vi "SetRtMode.vi"(8 "错误输入（无错误）":errorcluster, 10 "收发模式":u8) -> (0 "错误输出":errorcluster)   [LabVIEW 2018]
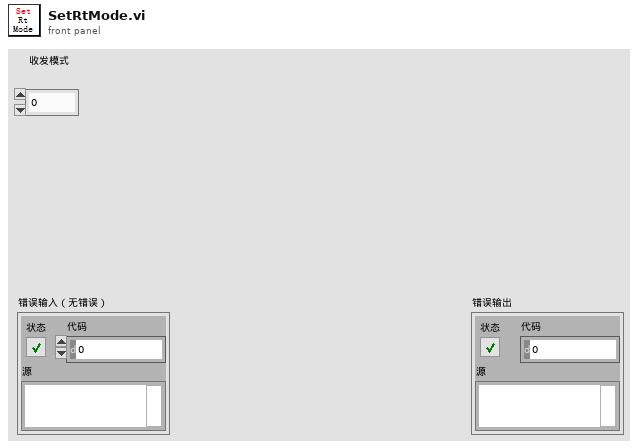
[diagram p1: front panel]
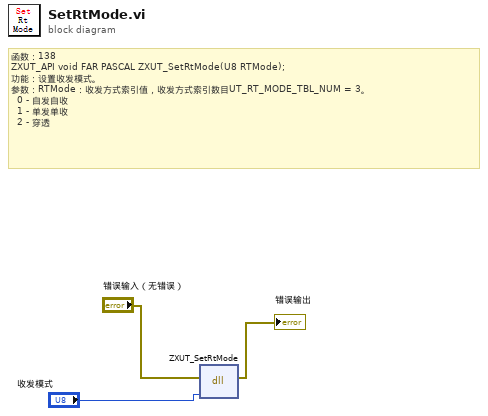
[diagram p0: block diagram]
diagram:
  # "函数：138\nZXUT_API void\tFAR PASCAL ZXUT_SetRtMode(U8 RTMode);\n功能：设置收发模式。\n参数：RTMode：收发方式索引值，收发方式索引数目UT_RT_MODE_TBL_NUM = 3。\n\t\t0 - 自发自收\n\t\t1 - 单发单收\n\t\t2 - 穿透"
  n1 = dll-call lib="PTH2Rabs E软件项目超声超声子VI函数VI\tTCG处理ZXUTConfigMgr.dll" fn="ZXUT_SetRtMode"(error in="错误输入（无错误）", "RTMode"="收发模式") -> (error out=→"错误输出":errorcluster)  [unwired: 4 in, 1 out]
